vi "DisableCache VxWorks.vi"(8 "error in (no error)":errorcluster, 11 "Cache Type":enum16{"_INSTRUCTION_CACHE", "_DATA_CACHE"}(ring)) -> (0 "error out":errorcluster, 3 "Status":u32)   [LabVIEW 2014]
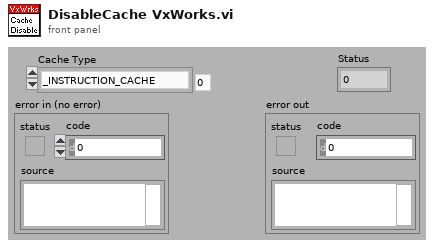
[diagram p1: front panel]
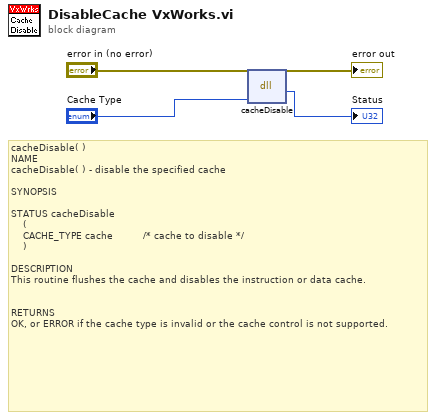
[diagram p0: block diagram]
diagram:
  # "cacheDisable( )\nNAME\ncacheDisable( ) - disable the specified cache\n\nSYNOPSIS\n\nSTATUS cacheDisable\n    (\n    CACHE_TYPE cache          /* cache to disable */\n    )\n\nDESCRIPTION\nThis routine flushes the cache and disables the instruction or data cache. \n\n\nRETURNS\nOK, or ERROR if the cache type is invalid or the cache control is not supported."
  n1 = dll-call lib="LabVIEW" fn="cacheDisable" ("vxWorks:cacheInvalidate")("Cache_Type"="Cache Type") -> ("Status"=→"Status":u32)  [unwired: 4 in, 2 out]
  "error out" <- "error in (no error)"
